vi "time-sec-to-time-str-RA.vi"(1 "Numeric":dbl format="%.2f") -> (0 "formatted-str":string)   [LabVIEW 2019]
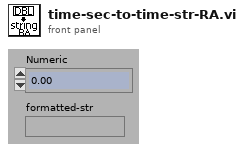
[diagram p1: front panel]
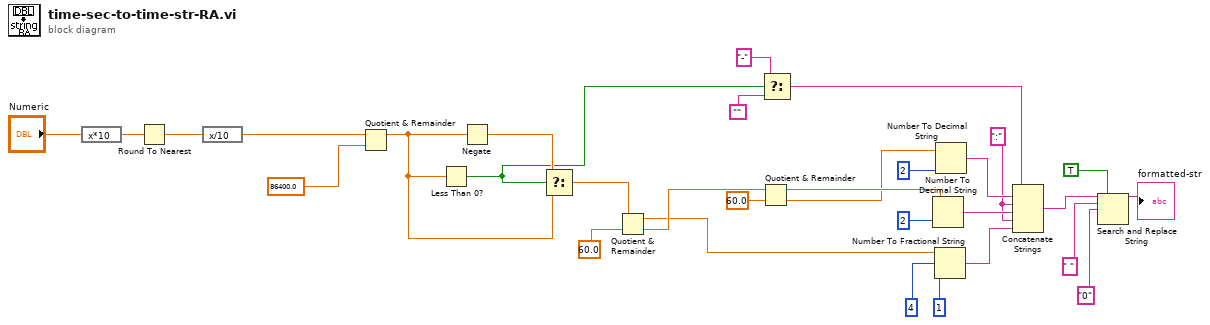
[diagram p0: block diagram]
diagram:
  w22 = ":" ("string")
  n1 = expression code="x*10"("Numeric") -> (w3:dbl)
  n2 = Round To Nearest(number=w3) -> (nearest integer value=w2:dbl)
  n3 = expression code="x/10"(w2) -> (w1:dbl)
  n4 = Quotient & Remainder(x=w1, y=86400.0) -> (x-y*floor(x/y)=w5:dbl)  [unwired: 1 out]
  n5 = Less Than 0?(x=w5) -> (x < 0?=w15:bool)
  n6 = Negate(x=w5) -> (-x=w17:dbl)
  n7 = Select(t=w17, s=w15, f=w5) -> (s? t:f=w16:dbl)
  n8 = Quotient & Remainder(x=w16, y=60.0) -> (x-y*floor(x/y)=w19:dbl, floor(x/y)=w21:dbl)
  n9 = Quotient & Remainder(x=w21, y=60.0) -> (x-y*floor(x/y)=w18:dbl, floor(x/y)=w14:dbl)
  n10 = Select(t="-" ("string"), s=w15, f="") -> (s? t:f=w13:string)
  n11 = Number To Decimal String(number=w18, width (-)=i16 2) -> (decimal integer string=w28:string)
  n12 = Number To Fractional String(number=w19, width (-)=i16 4, precision (6)=i16 1) -> (F-format string=w27:string)  [unwired: 1 in]
  n13 = Number To Decimal String(number=w14, width (-)=i16 2) -> (decimal integer string=w29:string)
  n14 = Concatenate Strings(w13, w29, w22, w28, w22, w27) -> (w26:string)
  n15 = Search and Replace String(replace all?=TRUE ("replace all? (F)"), input string=w26, search string=" ", replace string="0" ("replace string (\"\")")) -> (result string=→"formatted-str":string)  [unwired: 4 in, 3 out]
